vi "Get Status.vi"(8 "error in (no error)":errorcluster, 11 "Filter Wheel Simulator in":refnum<class "Filter Wheel Simulator.lvclass">) -> (0 "error out":errorcluster, 2 "FW Status":T1={"State"=enum."Move Complete", "Positions"=[], "Names"=[], "Notch"=[], "Moving"=[FALSE, FALSE]}, 3 "Filter Wheel Simulator out":refnum<class "Filter Wheel Simulator.lvclass">)   [LabVIEW 2024, in "Filter Wheel Simulator.lvclass"]
uses:
  Filter Wheel Simulator.lvclass
  FW cluster Status.ctl
  FW enum status.ctl
  Filter Wheel Object/Filter Wheel.lvclass
  Filter Wheel Simulator.lvclass/Filter Wheel Simulator.ctl
  Filter Wheel Object/Filter Wheel.lvclass/Filter Wheel.ctl
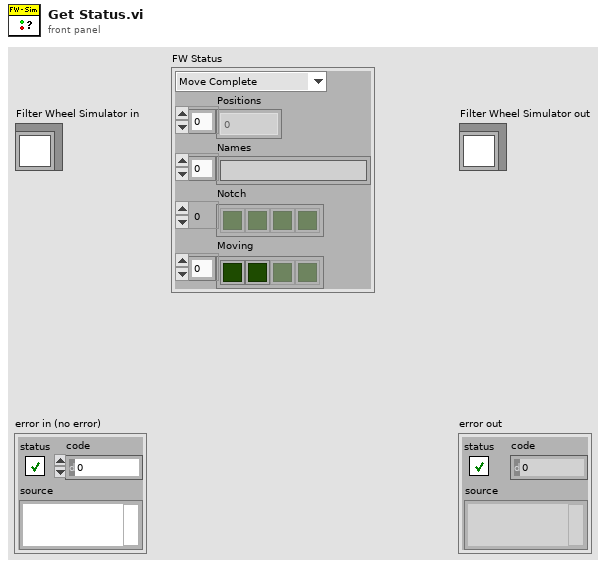
[diagram p1: front panel]
types:
  T1 = typedef "FW cluster Status.ctl" = cluster{"State":T2, "Positions":i32[], "Names":string[], "Notch":bool[], "Moving":bool[]}
  T2 = typedef "FW enum status.ctl" = enum16{"Initializing", "Moving", "Move Complete", "Error"}
  T3 = typedef "Filter Wheel Simulator.lvclass/Filter Wheel cluster Simulated Status.ctl" = cluster{"Move Start Time":timestamp, "Moving?":bool, "Target Pos":dbl, "Direction":bool}
  T4 = typedef "Filter Wheel Simulator.lvclass/Filter Wheel Move cluster.ctl" = cluster{"Wheel":i32, "Target Pos":i32}
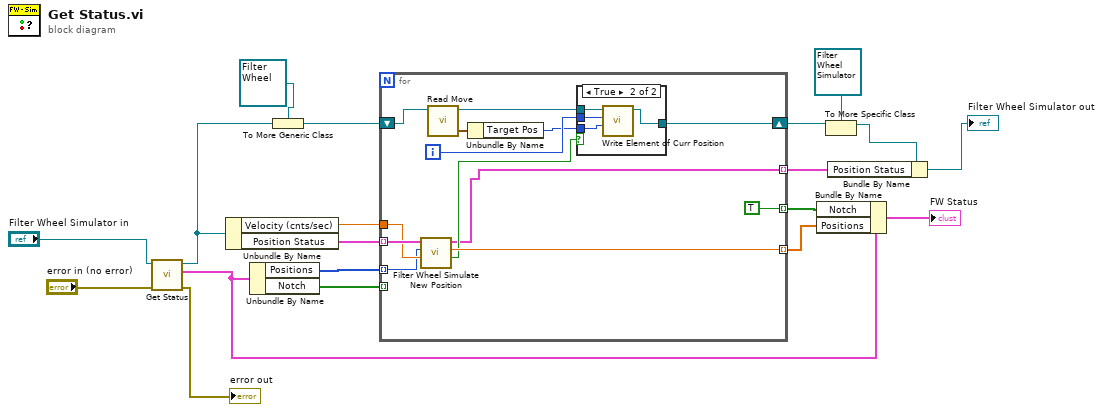
[diagram p0: block diagram]
diagram:
  n1 = call-parent "Get Status.vi"("error in (no error)"="error in (no error)", "Filter Wheel in"="Filter Wheel Simulator in") -> ("error out"=→"error out":errorcluster, "FW Status"=w13:T1, "Filter Wheel out"=w8:refnum<class "Filter Wheel Simulator.lvclass">)  [unwired: 7 in]
  n2 = Unbundle By Name(w8) -> ("Velocity (cnts/sec)"=w16:dbl, "Position Status"=w17:T3[])
  n3 = Unbundle By Name(w13) -> ("Positions"=w15:i32[], "Notch"=w14:bool[])
  n4 = To More Generic Class(target class=refnum<class "Filter Wheel.lvclass"> refnum ("Filter Wheel.lvclass"), reference=w8) -> (generic class reference=w6:refnum<class "Filter Wheel.lvclass">)
  n5 = for {
    tunnel: w17 -> [w32] mode=indexing
    tunnel: w16 -> [w31]
    tunnel: w15 -> [w30] mode=indexing
    tunnel: w14 -> [_] mode=indexing
    tunnel: [TRUE] -> w12 mode=indexing
    tunnel: [w29] -> w11 mode=indexing
    shift-right: [w22] -> w5
    shift-left: w6 -> [w27]
    tunnel: [w21] -> w2 mode=indexing
    i -> [w28]
    n6 = call "Filter Wheel Simulate New Position.vi"("Velocity (cnts/sec)"=w31, "Position"=w30, "Axis Status"=w32) -> ("move complete"=w24:bool, "New Pos"=w29:dbl, "Axis Status Out"=w21:T3)  [unwired: 6 in]
    n7 = call "Read Move.vi"("Filter Wheel in"=w27) -> ("Move"=w26:T4, "Filter Wheel out"=w25:refnum<class "Filter Wheel.lvclass">)  [unwired: 8 in, 1 out]
    n8 = Unbundle By Name(w26) -> ("Target Pos"=w23:i32)
    n9 = case shown="True" w24 {
      tunnel: w28 -> [_ w37]
      tunnel: w25 -> [w33 w36]
      tunnel: [w33 w35] -> w22
      tunnel: w23 -> [_ w34]
      frame False {
      }
      frame True {
        n10 = call "Write Element of Curr Position.vi"("Position idx"=w34, "Wheel"=w37, "Filter Wheel in"=w36) -> ("Filter Wheel out"=w35:refnum<class "Filter Wheel.lvclass">)  [unwired: 7 in, 1 out]
      }
    }
  }
  n11 = Bundle By Name(cluster=w13, "Notch"=w12, "Positions"=w11) -> (→"FW Status":T1)
  n12 = To More Specific Class(target class=refnum<class "Filter Wheel Simulator.lvclass"> refnum ("Filter Wheel Simulator out"), reference=w5) -> (specific class reference=w3:refnum<class "Filter Wheel Simulator.lvclass">)  [unwired: 1 in, 1 out]
  n13 = Bundle By Name(cluster=w3, "Position Status"=w2) -> (→"Filter Wheel Simulator out":refnum<class "Filter Wheel Simulator.lvclass">)
